vi "AWS-S3-BucketCreate.vi"(0 "AWS-S3-API":refnum<class "AWS-S3-API.lvclass">, 5 "Bucket Name":string, 7 "Versioning":enum16{"Off", "Enabled", "Suspended"}(ring), 9 "Log Target Bucket Name (blank for no logging)":string, 11 "error in":errorcluster, 12 "Index Document (blank for no website config)":string) -> (4 "AWS-S3-API out":refnum<class "AWS-S3-API.lvclass">, 15 "error out":errorcluster)   [LabVIEW 2012, in "AWS-S3-API.lvclass"]
uses:
  AWS-S3-API.lvclass
  C:/Users/Jack/repo/aws/AWS-SDK/AWSSDK.dll
  repo/aws/AWS-SDK/AWSSDK.dll
panel:
  # "Inputs"
  # "Outputs"
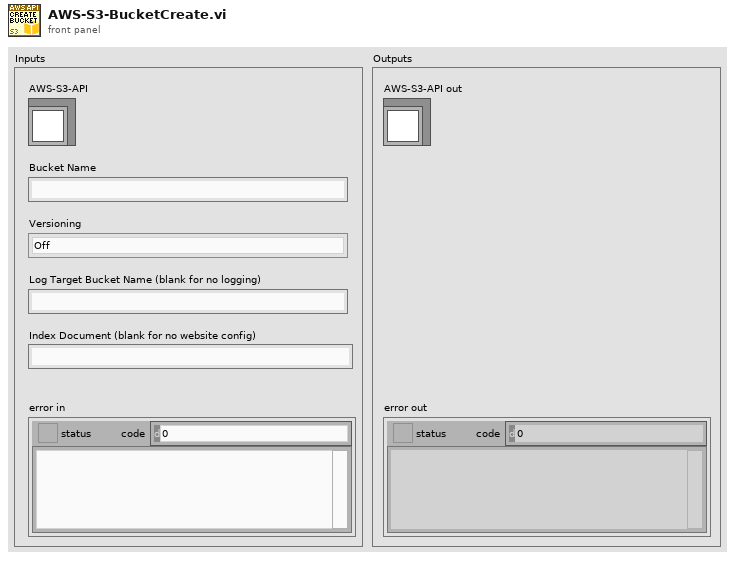
[diagram p1: front panel]
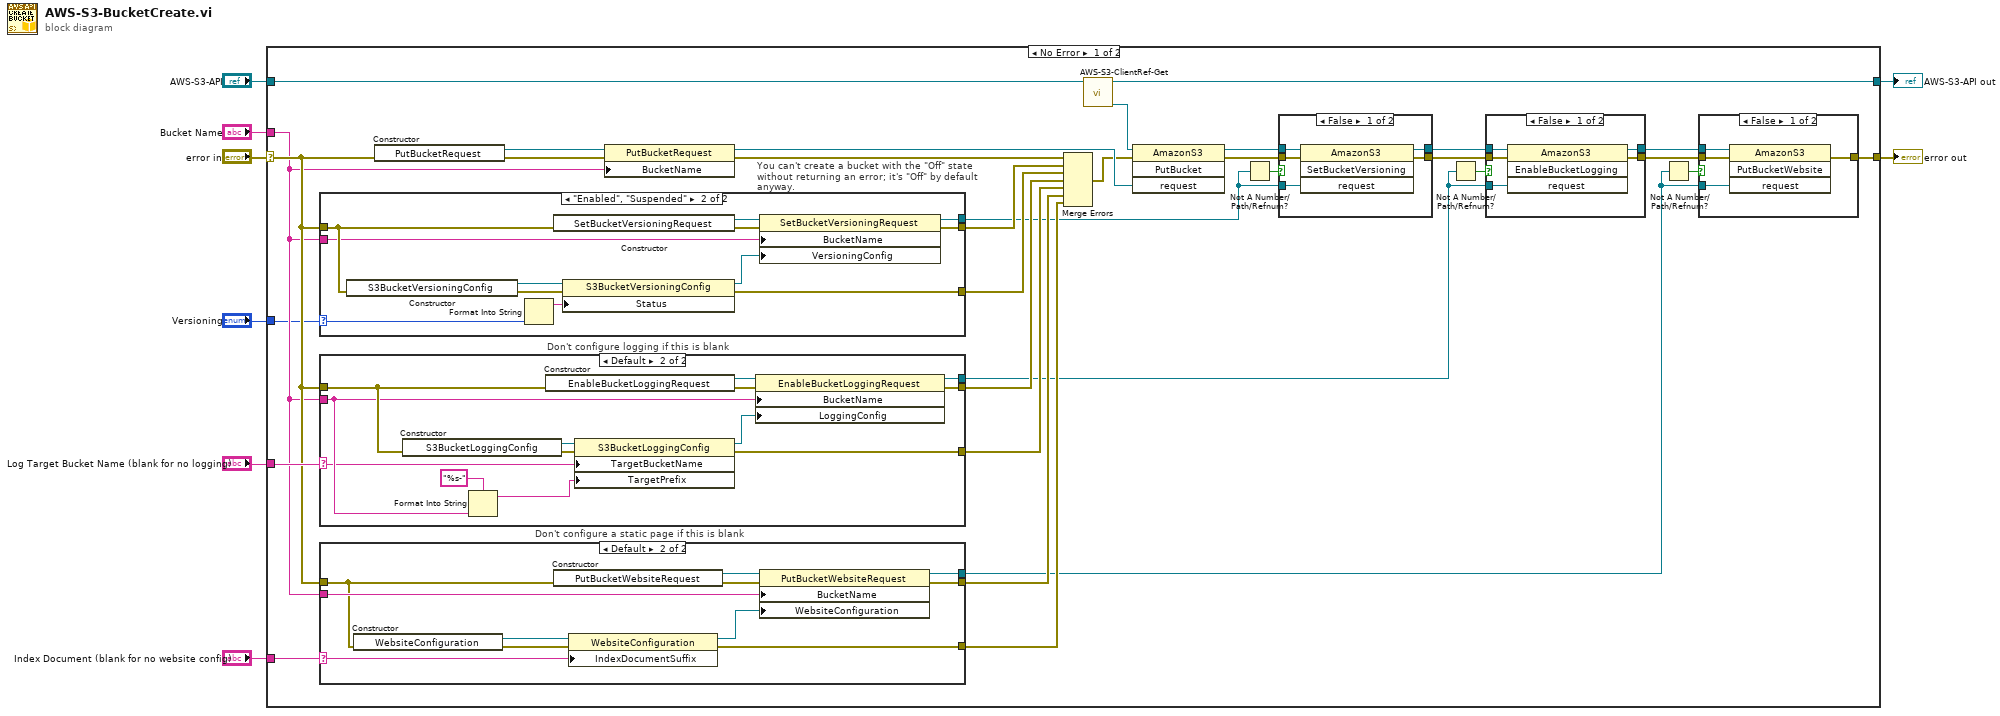
[diagram p0: block diagram]
diagram:
  n1 = case shown="No Error" "error in" {
    selector: "error in" -> [w24 w100]
    tunnel: [w18 w100] -> w8
    tunnel: [w9 w99] -> w6
    tunnel: "AWS-S3-API" -> [w10 w99]
    tunnel: "Bucket Name" -> [w23 _]
    tunnel: "Versioning" -> [w12 _]
    tunnel: "Log Target Bucket Name (blank for no logging)" -> [w27 _]
    tunnel: "Index Document (blank for no website config)" -> [w22 _]
    frame No Error {
      n2 = case "You can't create a bucket with the \"Off\" state without returning an error; it's \"Off\" by default anyway." shown="\"Enabled\", \"Suspended\"" w12 {
        selector: w12 -> [_ w42]
        tunnel: [w41 w53] -> w38
        tunnel: [w41 w52] -> w37
        tunnel: w24 -> [w41 w45]
        tunnel: w23 -> [_ w44]
        tunnel: [_ w43] -> w13
        frame "Off" {
        }
        frame "Enabled", "Suspended" {
          n3 = constructor class="S3BucketVersioningConfig"(error in=w45) -> (reference out=w51:refnum<k24>, error out=w48:errorcluster)  [unwired: 2 in, 1 out]
          n4 = Format Into String(w42) -> (resulting string=w47:string)  [unwired: 3 in, 1 out]
          n5 = constructor class="SetBucketVersioningRequest"(error in=w45) -> (reference out=w50:refnum<k24>, error out=w49:errorcluster)  [unwired: 2 in, 1 out]
          n6 = property class="S3BucketVersioningConfig"(reference=w51, error in=w48, "Status"=w47) -> (reference out=w46:refnum<k24>, error out=w52:errorcluster)
          n7 = property class="SetBucketVersioningRequest"(reference=w50, error in=w49, "BucketName"=w44, "VersioningConfig"=w46) -> (reference out=w43:refnum<k24>, error out=w53:errorcluster)
        }
      }
      n8 = case "Don't configure logging if this is blank" shown="Default" w27 {
        selector: w27 -> [_ w86]
        tunnel: [w85 w98] -> w36
        tunnel: [w85 w97] -> w35
        tunnel: w24 -> [w85 w90]
        tunnel: w23 -> [_ w89]
        tunnel: [_ w87] -> w26
        frame "" {
        }
        frame Default {
          n9 = constructor class="S3BucketLoggingConfig"(error in=w90) -> (reference out=w94:refnum<k24>, error out=w93:errorcluster)  [unwired: 2 in, 1 out]
          n10 = Format Into String(format string="%s-", w89) -> (resulting string=w91:string)  [unwired: 2 in, 1 out]
          n11 = constructor class="EnableBucketLoggingRequest"(error in=w90) -> (reference out=w96:refnum<k24>, error out=w95:errorcluster)  [unwired: 2 in, 1 out]
          n12 = property class="S3BucketLoggingConfig"(reference=w94, error in=w93, "TargetBucketName"=w86, "TargetPrefix"=w91) -> (reference out=w88:refnum<k24>, error out=w97:errorcluster)
          n13 = property class="EnableBucketLoggingRequest"(reference=w96, error in=w95, "BucketName"=w89, "LoggingConfig"=w88) -> (reference out=w87:refnum<k24>, error out=w98:errorcluster)
        }
      }
      n14 = case "Don't configure a static page if this is blank" shown="Default" w22 {
        selector: w22 -> [_ w71]
        tunnel: w24 -> [w66 w70]
        tunnel: w23 -> [_ w72]
        tunnel: [w66 w69] -> w40
        tunnel: [w66 w68] -> w39
        tunnel: [_ w67] -> w17
        frame "" {
        }
        frame Default {
          n15 = constructor class="WebsiteConfiguration"(error in=w70) -> (reference out=w73:refnum<k24>, error out=w76:errorcluster)  [unwired: 2 in, 1 out]
          n16 = constructor class="PutBucketWebsiteRequest"(error in=w70) -> (reference out=w74:refnum<k24>, error out=w75:errorcluster)  [unwired: 2 in, 1 out]
          n17 = property class="WebsiteConfiguration"(reference=w73, error in=w76, "IndexDocumentSuffix"=w71) -> (reference out=w77:refnum<k24>, error out=w68:errorcluster)
          n18 = property class="PutBucketWebsiteRequest"(reference=w74, error in=w75, "BucketName"=w72, "WebsiteConfiguration"=w77) -> (reference out=w67:refnum<k24>, error out=w69:errorcluster)
        }
      }
      n19 = constructor class="PutBucketRequest"(error in=w24) -> (reference out=w15:refnum<k24>, error out=w34:errorcluster)  [unwired: 2 in, 1 out]
      n20 = property class="PutBucketRequest"(reference=w15, error in=w34, "BucketName"=w23) -> (reference out=w33:refnum<k24>, error out=w31:errorcluster)
      n21 = Merge Errors(w31, w38, w37, w36, w35, w40, w39) -> (w30:errorcluster)
      n22 = call "AWS-S3-ClientRef-Get.vi"("AWS-S3-API"=w10) -> ("S3 Client ref"=w11:refnum<k24>, "AWS-S3-API out"=w9:refnum<class "AWS-S3-API.lvclass">)  [unwired: 9 in]
      n23 = invoke class="AmazonS3" method="PutBucket"(reference=w11, error in=w30, "request"=w33) -> (reference out=w16:refnum<k24>, error out=w32:errorcluster)  [unwired: 1 in, 2 out]
      n24 = Not A Number/Path/Refnum?(number/path/refnum=w13) -> (NaN/Path/Refnum?=w14:bool)
      n25 = case shown="False" w14 {
        tunnel: w32 -> [w58 w59]
        tunnel: [w57 w60] -> w29
        tunnel: [w56 w59] -> w28
        tunnel: w16 -> [w55 w60]
        tunnel: w13 -> [w54 _]
        frame False {
          n26 = invoke class="AmazonS3" method="SetBucketVersioning"(reference=w55, error in=w58, "request"=w54) -> (reference out=w57:refnum<k24>, error out=w56:errorcluster)  [unwired: 1 in, 2 out]
        }
        frame True {
        }
      }
      n27 = Not A Number/Path/Refnum?(number/path/refnum=w26) -> (NaN/Path/Refnum?=w25:bool)
      n28 = case shown="False" w25 {
        tunnel: w29 -> [w82 w83]
        tunnel: w28 -> [w81 w84]
        tunnel: w26 -> [w80 _]
        tunnel: [w79 w84] -> w19
        tunnel: [w78 w83] -> w20
        frame False {
          n29 = invoke class="AmazonS3" method="EnableBucketLogging"(reference=w82, error in=w81, "request"=w80) -> (reference out=w78:refnum<k24>, error out=w79:errorcluster)  [unwired: 1 in, 2 out]
        }
        frame True {
        }
      }
      n30 = Not A Number/Path/Refnum?(number/path/refnum=w17) -> (NaN/Path/Refnum?=w21:bool)
      n31 = case shown="False" w21 {
        tunnel: w20 -> [w64 _]
        tunnel: w19 -> [w63 w65]
        tunnel: w17 -> [w62 _]
        tunnel: [w61 w65] -> w18
        frame False {
          n32 = invoke class="AmazonS3" method="PutBucketWebsite"(reference=w64, error in=w63, "request"=w62) -> (error out=w61:errorcluster)  [unwired: 1 in, 3 out]
        }
        frame True {
        }
      }
    }
    frame Error {
    }
  }
  "error out" <- w8
  "AWS-S3-API out" <- w6
